vi "Linear_transform_of_points.vi"(8 "Analogue In":dbl[][](array[numeric])) -> (0 "Analogue Out":dbl[][](array[numeric]))   [LabVIEW 2010]
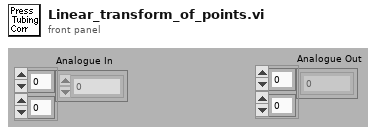
[diagram p1: front panel]
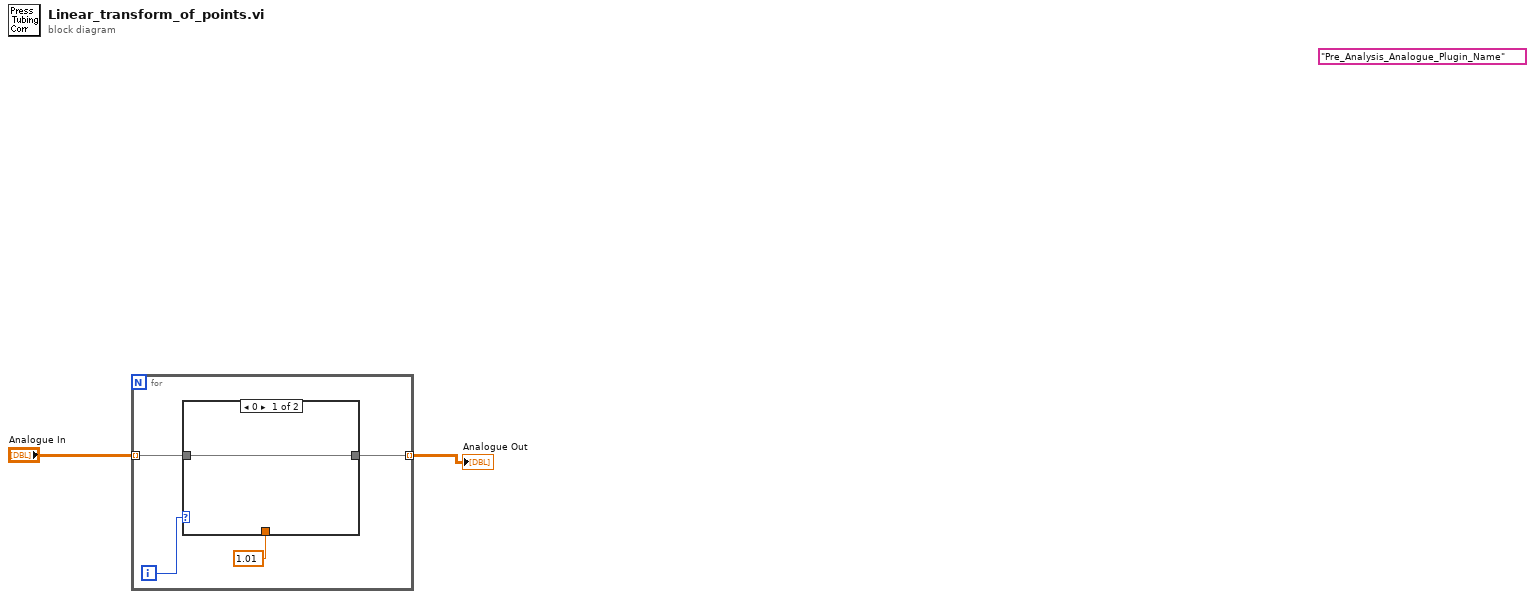
[diagram p0: block diagram]
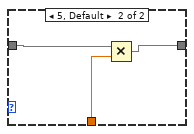
[diagram p2: hidden frame]
diagram:
  (unwired) "Pre_Analysis_Analogue_Plugin_Name"
  n1 = for {
    tunnel: [w5] -> w2 mode=indexing
    tunnel: "Analogue In" -> [w4] mode=indexing
    i -> [w6]
    n2 = case shown="0" w6 {
      tunnel: [w7 w9] -> w5
      tunnel: w4 -> [w7 w10]
      tunnel: 1.01 -> [_ w8]
      frame 0 {
      }
      frame 5, Default {
        n3 = Multiply(x=w10, y=w8) -> (x*y=w9:dbl[])
      }
    }
  }
  "Analogue Out" <- w2
